vi "refreshScriptRunList.vi"(8 "error in (no error)":errorcluster, 11 "ExperimentRunner in":refnum<class "ExperimentRunner.lvclass">) -> (0 "error out":errorcluster, 3 "ExperimentRunner out":refnum<class "ExperimentRunner.lvclass">)   [LabVIEW 2009, in "Views.lvlib" / "ExperimentControl.lvlib" / "ExperimentRunner.lvclass"]
uses:
  ExperimentRunner.lvclass
  ExperimentRunner.lvclass/ExperimentRunner.ctl
  Tools/Filing/FileSystem/FileSystem.lvclass
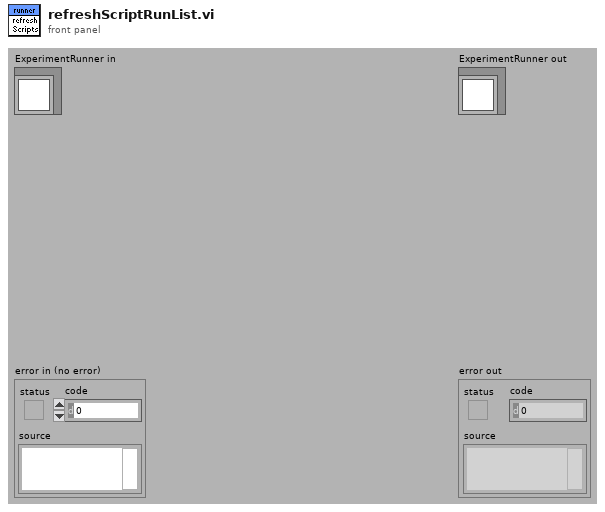
[diagram p1: front panel]
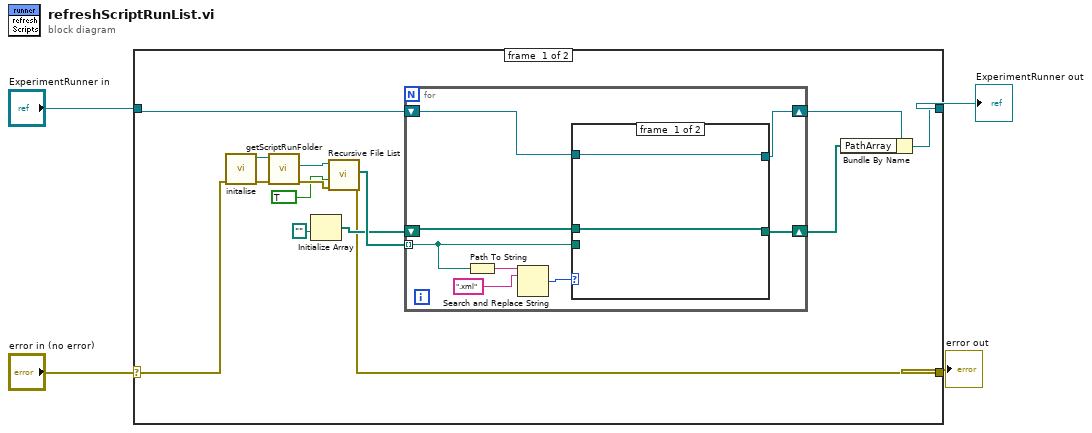
[diagram p0: block diagram]
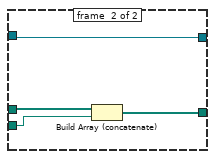
[diagram p2: hidden frame]
diagram:
  n1 = case shown="No Error" "error in (no error)" {
    selector: "error in (no error)" -> [w16 w34]
    tunnel: [w5 w34] -> w3
    tunnel: [w9 w33] -> w1
    tunnel: "ExperimentRunner in" -> [w14 w33]
    frame #0 {
      n2 = call "initalise.vi"("error in (no error)"=w16) -> ("error out"=w17:errorcluster, "FileSystem out"=w18:refnum<class "FileSystem.lvclass">)  [unwired: 9 in]
      n3 = call "getScriptRunFolder.vi"("error in (no error)"=w17, "FileSystem.lvclass in"=w18) -> ("error out"=w7:errorcluster, "ScriptRunFolder"=w15:path)  [unwired: 7 in, 1 out]
      n4 = Initialize Array(path "") -> (w12:path[])  [unwired: 1 in]
      n5 = call <vilib>:"Recursive File List.vi"("error in (no error)"=w7, "Continue Recursing on Error? (F)"=TRUE, "Folder Path"=w15) -> ("error out"=w5:errorcluster, "All Files in Dir"=w13:path[])  [unwired: 4 in, 3 out]
      n6 = for {
        tunnel: w13 -> [w22] mode=indexing
        shift-right: [w21] -> w8
        shift-left: w12 -> [w23]
        shift-right: [w19] -> w10
        shift-left: w14 -> [w20]
        n7 = Path To String(path=w22) -> (string=w26:string)
        n8 = Search and Replace String(input string=w26, search string=".xml") -> (number of replacements=w24:i32)  [unwired: 6 in, 3 out]
        n9 = case shown="1, Default" w24 {
          tunnel: w23 -> [w28 w32]
          tunnel: w22 -> [_ w29]
          tunnel: [w28 w31] -> w21
          tunnel: w20 -> [w27 w30]
          tunnel: [w27 w30] -> w19
          frame #0 {
          }
          frame #1 {
            n10 = Build Array (concatenate)(w32, w29) -> (w31:path[])
          }
        }
      }
      n11 = Bundle By Name(cluster=w10, "PathArray"=w8) -> (w9:refnum<class "ExperimentRunner.lvclass">)
    }
    frame #1 {
    }
  }
  "error out" <- w3
  "ExperimentRunner out" <- w1
